vi "Read Command.vi"(8 "error in (no error)":errorcluster, 11 "TI in":refnum<class "TI.lvclass">) -> (0 "error out":errorcluster, 2 "read buffer":string, 3 "TI out":refnum<class "TI.lvclass">)   [LabVIEW 2020, in "TI.lvclass"]
uses:
  TI.lvclass
  Abstract/Serial Device/Serial Device.lvclass
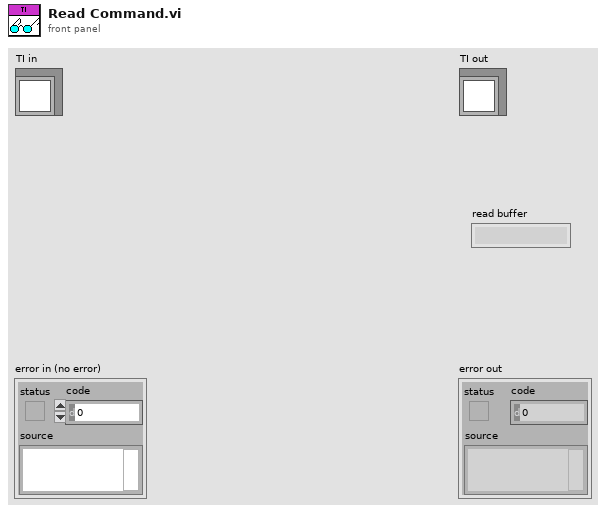
[diagram p1: front panel]
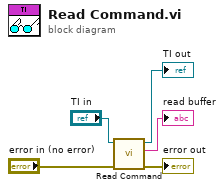
[diagram p0: block diagram]
diagram:
  n1 = call-parent "Read Command.vi"("error in (no error)"="error in (no error)", "Serial Device in"="TI in") -> ("error out"=→"error out":errorcluster, "read buffer"=→"read buffer":string, "Serial Device out"=→"TI out":refnum<class "TI.lvclass">)  [unwired: 7 in]
